vi "dataSplitter.vi"(3 "Input":string) -> (0 "After \\t":string, 1 "Before \\t":string)   [LabVIEW 2019]
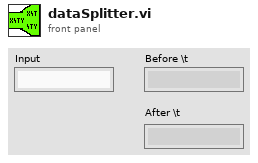
[diagram p1: front panel]
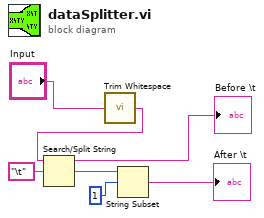
[diagram p0: block diagram]
diagram:
  n1 = call <vilib>:"Trim Whitespace.vi"("string"="Input") -> ("trimmed string"=w1:string)  [unwired: 1 in]
  n2 = Search/Split String(string=w1, search string/char (-)="\t") -> (substring before match=→"Before \\t":string, match + rest of string=w5:string)  [unwired: 1 in, 1 out]
  n3 = String Subset(string=w5, offset (0)=1) -> (substring=→"After \\t":string)  [unwired: 1 in]
